vi "Write VISA session.vi"(8 "error in (no error)":errorcluster, 10 "VISA session":refnum<visa-resource-name>, 11 "Scope VISA CFG in":refnum<class "Scope VISA CFG.lvclass">) -> (0 "error out":errorcluster, 3 "Scope VISA CFG out":refnum<class "Scope VISA CFG.lvclass">)   [LabVIEW 2023, in "Scope VISA.lvlib" / "Scope VISA CFG.lvclass"]
uses:
  Scope VISA CFG.lvclass
  Scope VISA CFG.lvclass/Scope VISA CFG.ctl
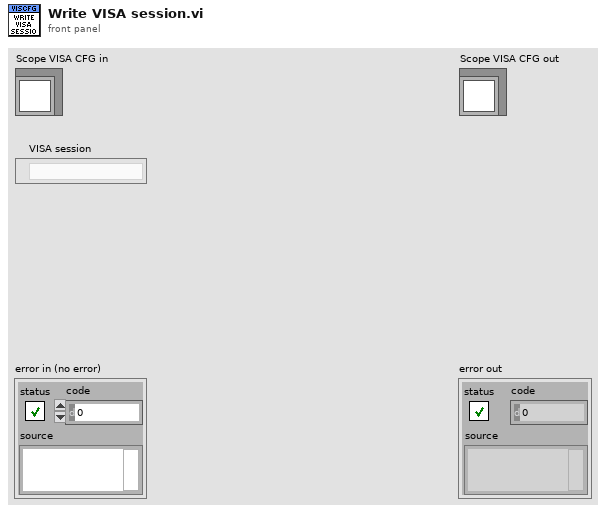
[diagram p1: front panel]
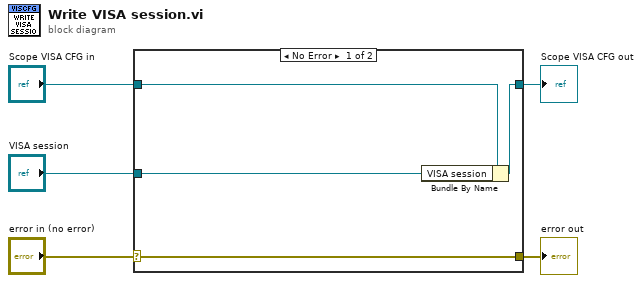
[diagram p0: block diagram]
diagram:
  n1 = case shown="No Error" "error in (no error)" {
    selector: "error in (no error)" -> [w9 w10]
    tunnel: [w9 w10] -> w4
    tunnel: [w7 w11] -> w2
    tunnel: "Scope VISA CFG in" -> [w8 w11]
    tunnel: "VISA session" -> [w6 _]
    frame No Error {
      n2 = Bundle By Name(cluster=w8, "VISA session"=w6) -> (w7:refnum<class "Scope VISA CFG.lvclass">)
    }
    frame Error {
    }
  }
  "error out" <- w4
  "Scope VISA CFG out" <- w2
